vi "BotCOMCntrlPanel.vi"() -> ()   [LabVIEW 2014]
uses:
  <userlib>/botspeak/VIs/SubVIs/BotSpeak_Globals.vi
  <userlib>/botspeak/VIs/Direct/BotSpeak_Control.ctl
panel:
  out "Array":string[](array[string])
  out "VIs running":i16
  out "Status String":string
  out "Talking":bool
  out "Status":string
  out "reply":T2
  out "send":T3
  in  "stop":bool
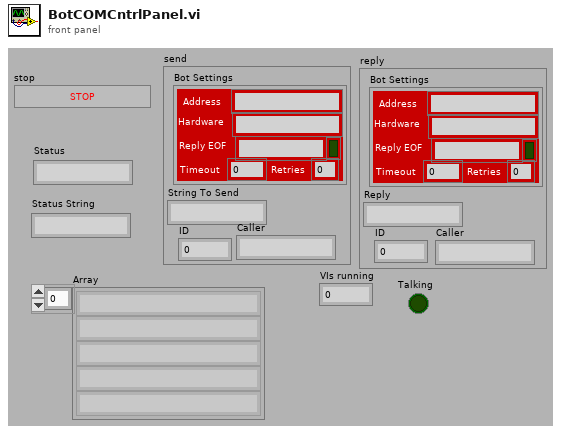
[diagram p1: front panel]
types:
  T1 = typedef "BotSpeak_Control.ctl" = cluster{"Address":string, "Reply EOF":string, "Hardware":string, "Retries":i8, "Timeout":i32, "Open?":bool}
  T2 = cluster{"Bot Settings":T1, "Reply":string, "ID":dbl, "Caller":string}
  T3 = cluster{"Bot Settings":T1, "String To Send":string, "ID":dbl, "Caller":string}
  T4 = enum32{"Bad", "Idle", "Run top level", "Running"}
  T5 = cluster{"Bot Settings":T1, "String":string, "ID":dbl, "Caller":string}
  T6 = typedef "CommState.ctl" = cluster{"Bot Settings":T1, "Initialized":bool, "Talking":bool}
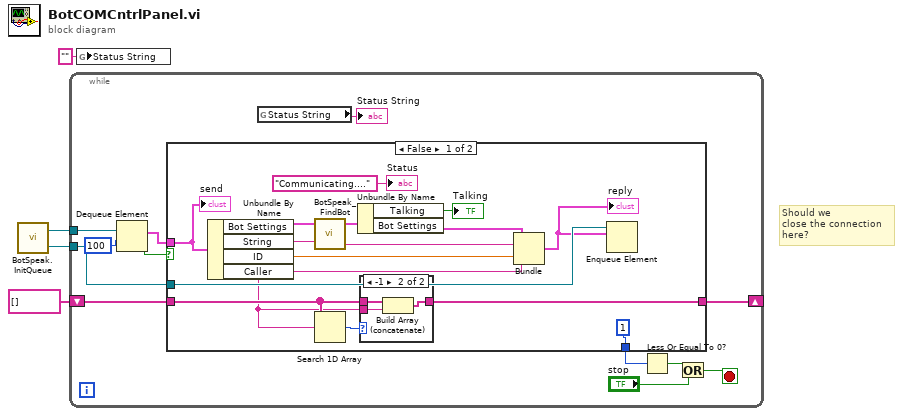
[diagram p0: block diagram]
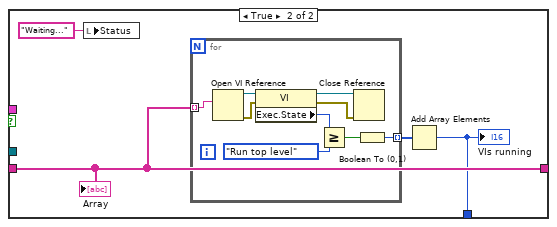
[diagram p3: hidden frame]
diagram:
  # "Should we \nclose the connection\nhere?"
  n1 = call <userlib>:"BotSpeak.InitQueue.vi"() -> ("ReadQueue"=w3:refnum<queue>, "SendQueue"=w4:refnum<queue>)  [unwired: 2 in]
  n2 = while {
    tunnel: w4 -> [w16]
    tunnel: w3 -> [w14]
    shift-right: [w5] -> _
    shift-left: string[] [] -> [w6]
    stop <- w9 stop-if-true
    n3 = Dequeue Element(queue=w16, timeout in ms (-1)=100) -> (element=w15:T5, timed out?=w12:bool)  [unwired: 1 in, 2 out]
    n4 = case shown="False" w12 {
      tunnel: w15 -> [w24 _]
      tunnel: w14 -> [w29 _]
      tunnel: [i16 1 w37] -> w7
      tunnel: w6 -> [w19 w38]
      tunnel: [w17 w38] -> w5
      frame False {
        n5 = Unbundle By Name(w24) -> ("Bot Settings"=w30:T1, "String"=w32:string, "ID"=w28:dbl, "Caller"=w18:string)
        n6 = call <userlib>:"BotSpeak_FindBot.vi"("String To Send"=w32, "Bot Settings"=w30) -> ("Reply"=w31:string, "Connection"=w25:T6)  [unwired: 1 in, 1 out]
        n7 = Search 1D Array(1D array=w19, element=w18) -> (index of element=w20:i32)  [unwired: 1 in]
        n8 = Unbundle By Name(w25) -> ("Talking"=→"Talking":bool, "Bot Settings"=w26:T1)
        n9 = case shown="-1" w20 {
          tunnel: w19 -> [w33 w36]
          tunnel: w18 -> [_ w35]
          tunnel: [w33 w34] -> w17
          frame Default {
          }
          frame -1 {
            n10 = Build Array (concatenate)(w36, w35) -> (w34:string[])
          }
        }
        n11 = Bundle("Bot Settings"=w26, "Reply"=w31, "ID"=w28, "Caller"=w18) -> (w27:T2)  [unwired: 1 in]
        "reply" <- w27
        n12 = Enqueue Element(queue=w29, element=w27) -> ()  [unwired: 2 in, 3 out]
        "send" <- w24
        "Status" <- "Communicating...." ("Status")
      }
      frame True {
        n13 = local write "Status"("Waiting..." ("Status")) -> ()
        n14 = for {
          tunnel: [w42] -> w39 mode=indexing
          tunnel: w38 -> [w41] mode=indexing
          n15 = Open VI Reference(vi path=w41) -> (vi reference=w49:refnum<vi>, error out=w48:errorcluster)  [unwired: 5 in]
          n16 = property class="VI"(reference=w49, error in=w48) -> (reference out=w44:refnum<vi>, error out=w45:errorcluster, "Exec.State"=w47:T4)
          n17 = Greater Or Equal?(x=w47, y=T4."Run top level") -> (x >= y?=w43:bool)
          n18 = Close Reference(reference=w44, error in (no error)=w45) -> ()  [unwired: 1 out]
          n19 = Boolean To (0,1)(Boolean=w43) -> (0, 1=w42:i16)
        }
        n20 = Add Array Elements(numeric array=w39) -> (sum=w37:i16)
        "VIs running" <- w37
        "Array" <- w38
      }
    }
    n21 = global read "BotSpeak_Globals.vi" "Status String"() -> (→"Status String":string)
    n22 = Less Or Equal To 0?(x=w7) -> (x <= 0?=w8:bool)
    n23 = Or(x=w8, y="stop") -> (x .or. y?=w9:bool)
  }
  n24 = global write "BotSpeak_Globals.vi" "Status String"("" ("Script Sent")) -> ()
